vi "HostOffsetWithdrawSimulator.vi"() -> ()   [LabVIEW 2014]
uses:
  <vilib>/FPGAPlugInAG/PCIe-7851R/niLvFpga_Open_PCIe-7851R.vi
  <vilib>/rvi/interface/common/dynamic/niFpgaDynamicAddResources.vi
  <vilib>/Utility/error.llb/Error Cluster From Error Code.vi
  <vilib>/rvi/errors/niLvFpgaAdjustHostInterfaceError.vi
  <vilib>/FPGAPlugInAG/Dynamic/niLvFpga_Close_Dynamic.vi
  <vilib>/rvi/interface/nirviOpenFPGA/nirviOpenFPGA.xnode
  FPGA Bitfiles/UntitledProject1_FPGATarget_FPGAOffsetWithdr_n0jCGoJhCm0.lvbitx
  <vilib>/rvi/interface/nirviReadWriteControl/nirviReadWriteControl.xnode
  <vilib>/rvi/interface/nirviMethod/nirviMethod.xnode
  <vilib>/rvi/interface/nirviCloseFPGA/nirviCloseFPGA.xnode
  <vilib>/FPGAPlugInAG/Dynamic/niLvFpga_ReadFifo_Dynamic.vi
  <vilib>/rvi/errors/niLvFpgaMergeErrorWithErrorCode.vi
  NiFpgaLv.dll
  <vilib>/rvi/interface/Simulation/niFpgaSimulationCallBeginRW.vi
panel:
  out "Elements Remaining":u32
  in  "stop":bool
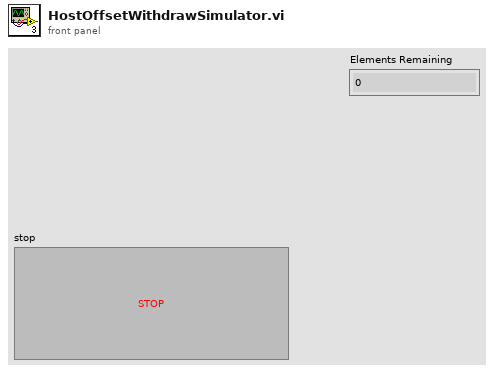
[diagram p1: front panel]
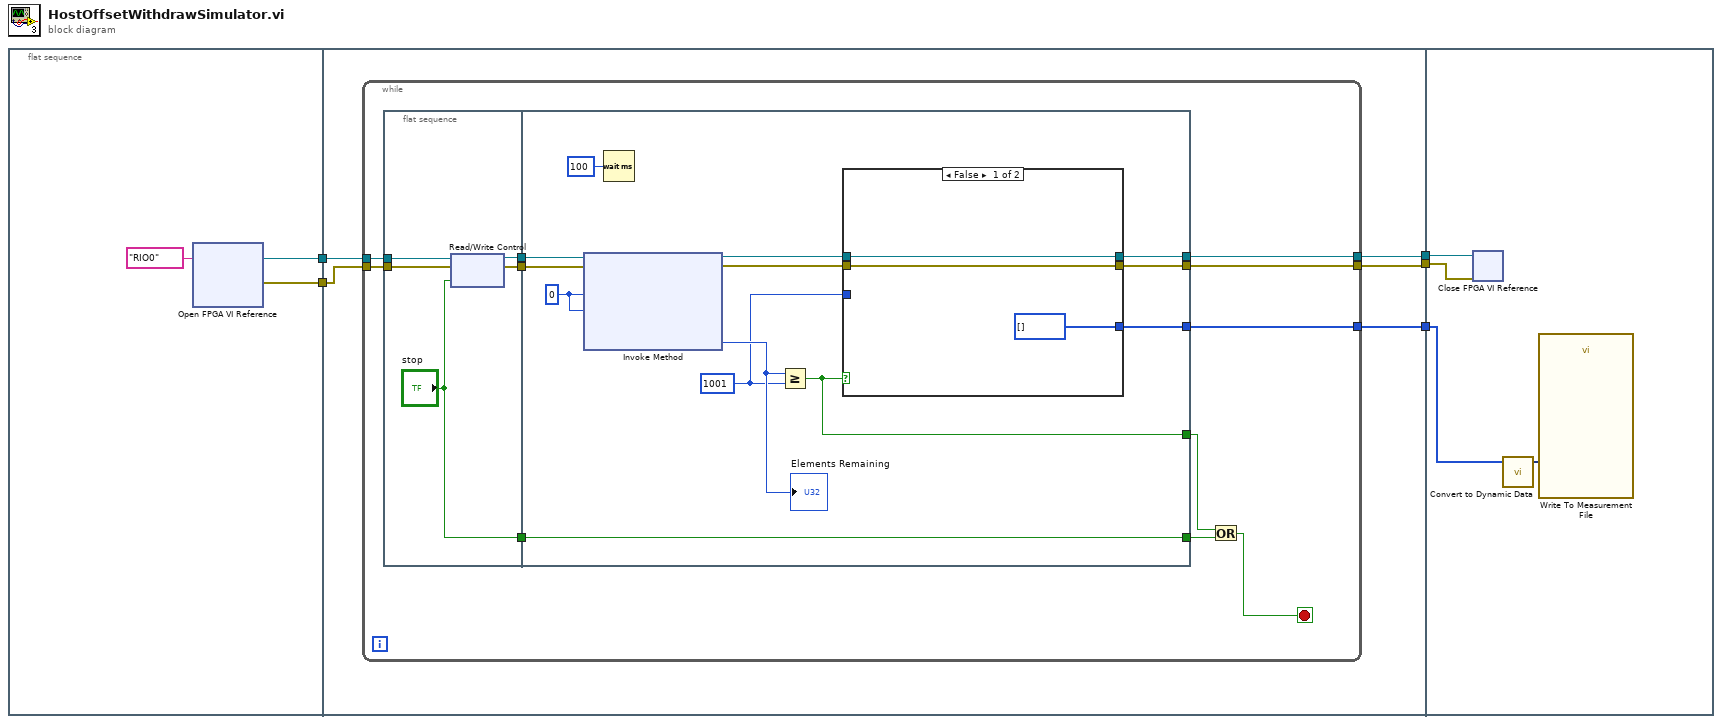
[diagram p0: block diagram]
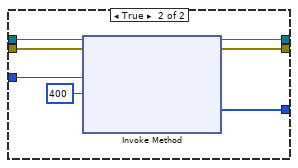
[diagram p2: hidden frame]
diagram:
  n1 = flat-sequence {
    tunnel: [w7] -> w5
    tunnel: [w6] -> w4
    tunnel: w5 -> [w13]
    tunnel: w4 -> [w12]
    tunnel: [w11] -> w3
    tunnel: [w10] -> w2
    tunnel: [w9] -> w1
    tunnel: w3 -> [w56]
    tunnel: w2 -> [w55]
    tunnel: w1 -> [w54]
    frame #0 {
      n2 = xnode "Open FPGA VI Reference"("resource name"=tag "RIO0") -> ("FPGA VI Reference Out"=w7:refnum<k20>, "error out"=w6:errorcluster)  [unwired: 1 in]
    }
    frame #1 {
      n3 = while {
        tunnel: w13 -> [w24]
        tunnel: w12 -> [w23]
        tunnel: [w20] -> w11
        tunnel: [w19] -> w10
        tunnel: [w18] -> w9
        stop <- w14 stop-if-true
        n4 = flat-sequence {
          tunnel: w24 -> [w29]
          tunnel: w23 -> [w28]
          tunnel: [w27] -> w22
          tunnel: [w26] -> w21
          tunnel: ["stop"] -> w17
          tunnel: w22 -> [w42]
          tunnel: w21 -> [w41]
          tunnel: [w35] -> w20
          tunnel: [w34] -> w19
          tunnel: [w33] -> w18
          tunnel: w17 -> [w31]
          tunnel: [w31] -> w16
          tunnel: [w30] -> w15
          frame #0 {
            n5 = xnode "Read/Write Control"("FPGA VI Reference In"=w29, "error in"=w28, "stop"="stop") -> ("FPGA VI Reference Out"=w27:refnum<k20>, "error out"=w26:errorcluster)
          }
          frame #1 {
            w32 = u32 1001 ("y")
            w39 = 0
            n6 = xnode "Invoke Method"("FPGA VI Reference In"=w42, "error in"=w41, "Number of Elements"=w39, "Timeout (ms)"=w39) -> ("FPGA VI Reference Out"=w37:refnum<k20>, "error out"=w36:errorcluster, "Elements Remaining"=w38:u32)  [unwired: 1 out]
            "Elements Remaining" <- w38
            n7 = Wait (ms)(milliseconds to wait=u32 100) -> ()  [unwired: 1 out]
            n8 = Greater Or Equal?(x=w38, y=w32) -> (x >= y?=w30:bool)
            n9 = case shown="False" w30 {
              tunnel: w37 -> [w45 w52]
              tunnel: w36 -> [w44 w51]
              tunnel: [w45 w50] -> w35
              tunnel: [w44 w49] -> w34
              tunnel: [i16[] [] ("Data") w48] -> w33
              tunnel: w32 -> [_ w47]
              frame False {
              }
              frame True {
                n10 = xnode "Invoke Method"("FPGA VI Reference In"=w52, "error in"=w51, "Number of Elements"=w47, "Timeout (ms)"=400) -> ("FPGA VI Reference Out"=w50:refnum<k20>, "error out"=w49:errorcluster, "Data"=w48:i16[])  [unwired: 1 out]
              }
            }
          }
        }
        n11 = Or(x=w15, y=w16) -> (x .or. y?=w14:bool)
      }
    }
    frame #2 {
      n12 = xnode "Close FPGA VI Reference"("FPGA VI Reference In"=w56, "error in"=w55) -> ()  [unwired: 1 out]
      n13 = call "Convert to Dynamic Data"("Array"=w54) -> ("Dynamic Data Type"=w53:dynamicdata)  [unwired: 3 in]
      n14 = call "Write To Measurement File"("Signals"=w53) -> ()  [unwired: 16 in, 3 out]
    }
  }
